vi "Main.vi"() -> ()   [LabVIEW 2017]
uses:
  System.Windows.Forms
panel:
  in  "Stop":bool
  in  "Button":refnum<k24>(container)
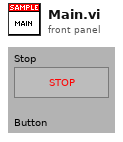
[diagram p1: front panel]
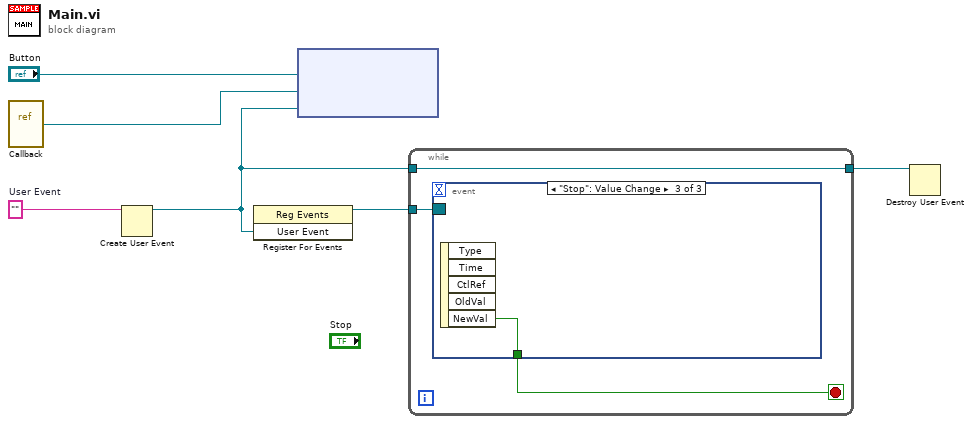
[diagram p0: block diagram]
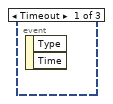
[diagram p2: hidden frame]
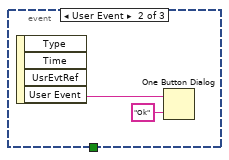
[diagram p3: hidden frame]
diagram:
  w5 = ""  # User Event
  n1 = vi-ref "Callback.vi"() -> ("vi reference"=w4:refnum<vi>)
  n2 = Create User Event(user event datatype=w5) -> (user event=w2:refnum<user-event>)  [unwired: 1 in, 1 out]
  n3 = register-events(w2) -> (reference out=w3:refnum<event-registration>)  [unwired: 2 in, 1 out]
  n4 = node("Button", w4, w2) -> ()  [unwired: 2 in, 2 out]
  n5 = while {
    tunnel: w3 -> [w9]
    tunnel: w2 -> [w7]
    tunnel: [w7] -> w1
    stop <- w8 stop-if-true
    n6 = event shown="[2] \"Stop\": Value Change" {
      selector: w9 -> [_ _ _]
      dyn-events: _ -> [_ _ _]
      timeout: _ -> [_ _ _]
      tunnel: [_ _ w12] -> w8
      event Timeout {
        n7 = event-data() -> ()  [unwired: 1 in, 2 out]
      }
      event User Event {
        n8 = event-data() -> ("User Event"=w11:string)  [unwired: 1 in, 3 out]
        n9 = One Button Dialog(message=w11, button name ("OK")="Ok") -> ()  [unwired: 1 out]
      }
      event "Stop": Value Change {
        n10 = event-data() -> ("NewVal"=w12:bool)  [unwired: 1 in, 4 out]
      }
    }
  }
  n11 = Destroy User Event(user event=w1) -> ()  [unwired: 1 in, 1 out]
